vi "Option.vi"(8 "error in":errorcluster, 10 "Test Result In":T3, 11 "CalCfg File In":T2) -> (0 "error out":errorcluster, 1 "Pass":bool, 2 "Test Result Out":T3, 3 "CalCfg File Out":T2, 4 "String":string)   [LabVIEW 2020, in "GUCalibration2.lvlib"]
uses:
  GUCalibration2.lvlib
  Controls/Test Result.ctl
  Controls/Site Data Element.ctl
  Controls/Site Raw Data Element.ctl
  Controls/CalibrationOrCheck.ctl
  Utilities/Read Key Boolean.vi
  Utilities/Write Key Path.vi
  Utilities/Write Key Boolean.vi
panel:
  in  "Cal/Check":T1
  in  "GU Bench File Path":path
  in  "Cancel":bool
  in  "OK":bool
  in  "Offset File Path":path
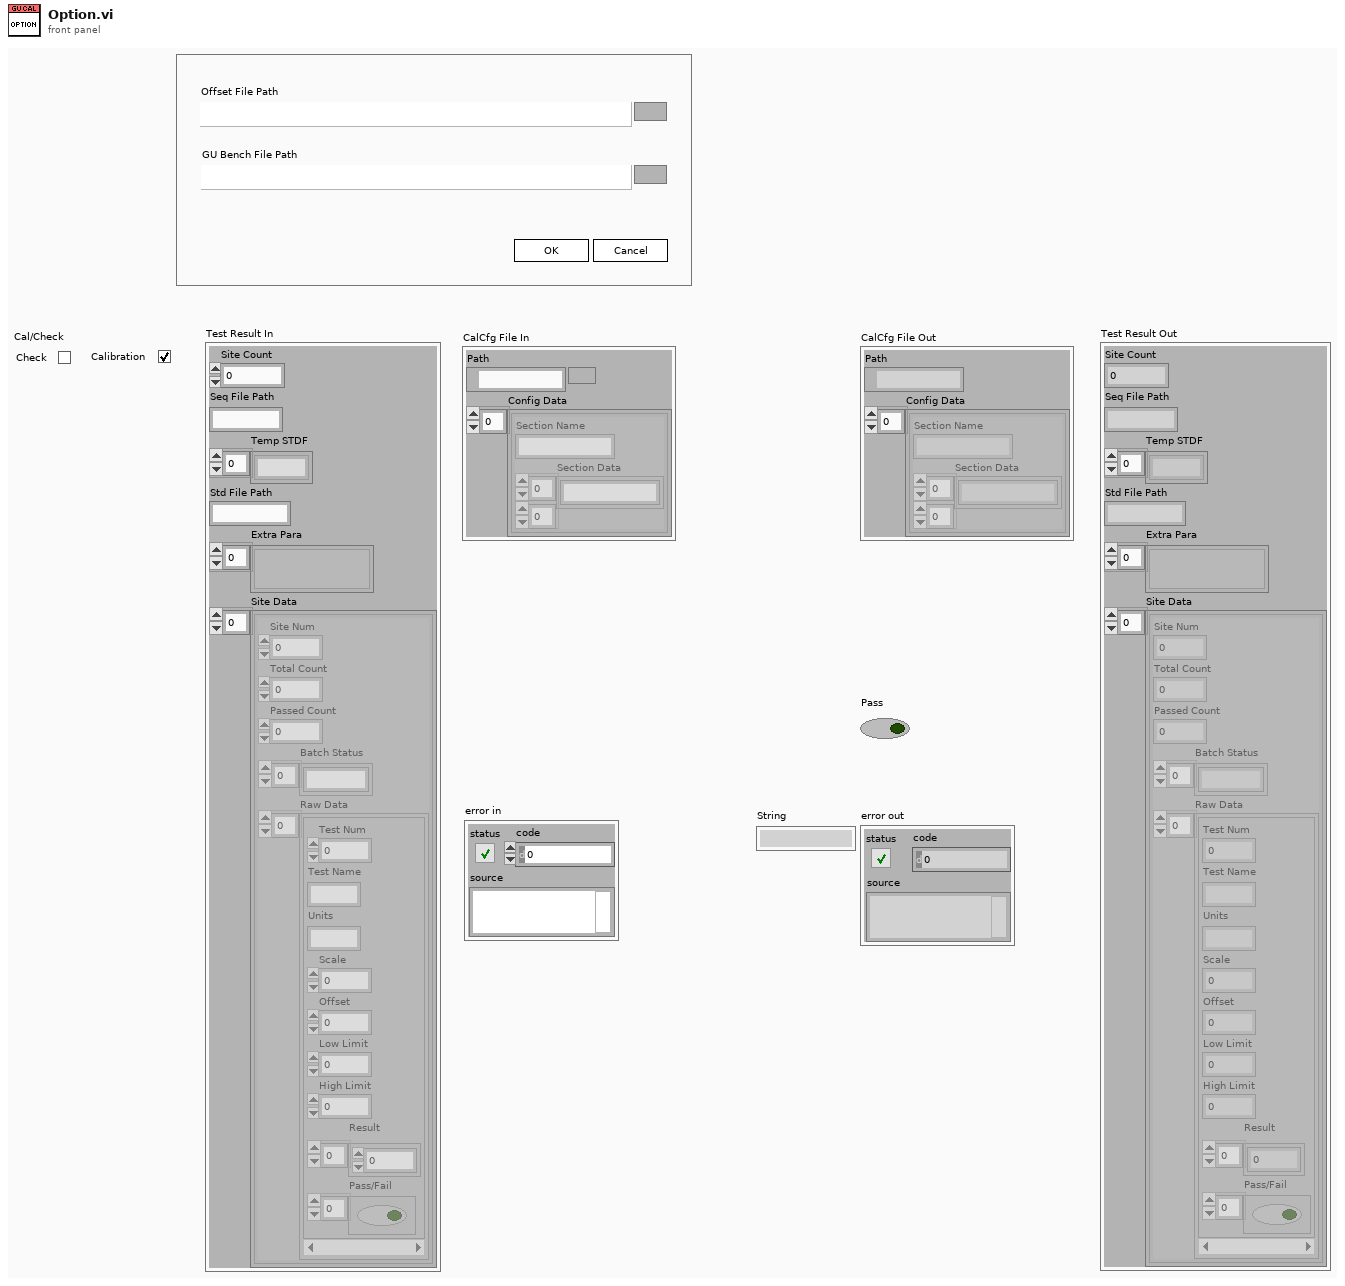
[diagram p1: front panel]
types:
  T1 = typedef "GUCalibration2.lvlib/CalibrationOrCheck.ctl" = enum32{"Calibration", "Check"}
  T2 = cluster{"Path":path, "Config Data":cluster{"Section Name":string, "Section Data":string[][]}[]}
  T3 = typedef "GUCalibration2.lvlib/Test Result.ctl" = cluster{"Site Count":i32, "Seq File Path":string, "Temp STDF":string[], "Std File Path":string, "Extra Para":variant[], "Site Data":T4[]}
  T4 = typedef "GUCalibration2.lvlib/Site Data Element.ctl" = cluster{"Site Num":i32, "Total Count":i32, "Passed Count":i32, "Batch Status":string[], "Raw Data":T5[]}
  T5 = typedef "GUCalibration2.lvlib/Site Raw Data Element.ctl" = cluster{"Test Num":u32, "Test Name":string, "Units":string, "Scale":i8, "Offset":dbl, "Low Limit":dbl, "High Limit":dbl, "Result":dbl[], "Pass/Fail":bool[]}
  T6 = cluster{"Section Name":string, "Section Data":string[][]}[]
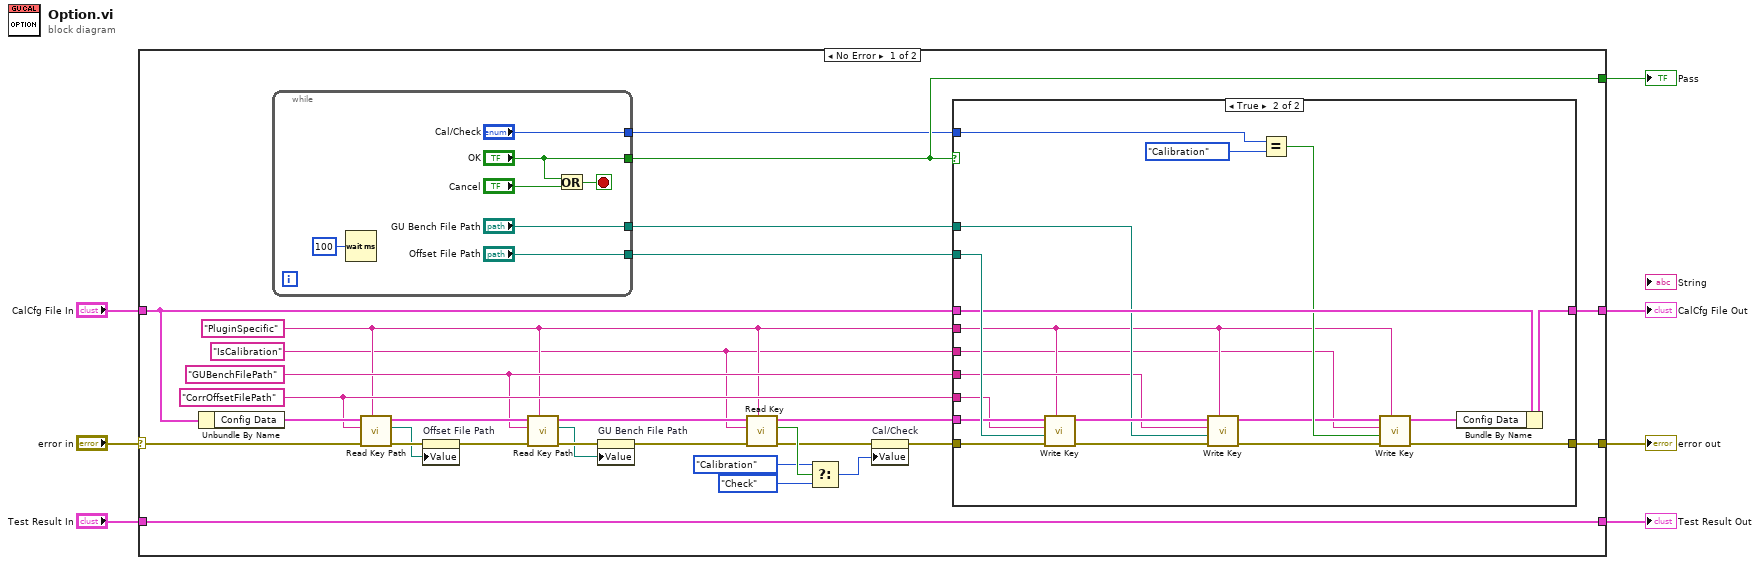
[diagram p0: block diagram]
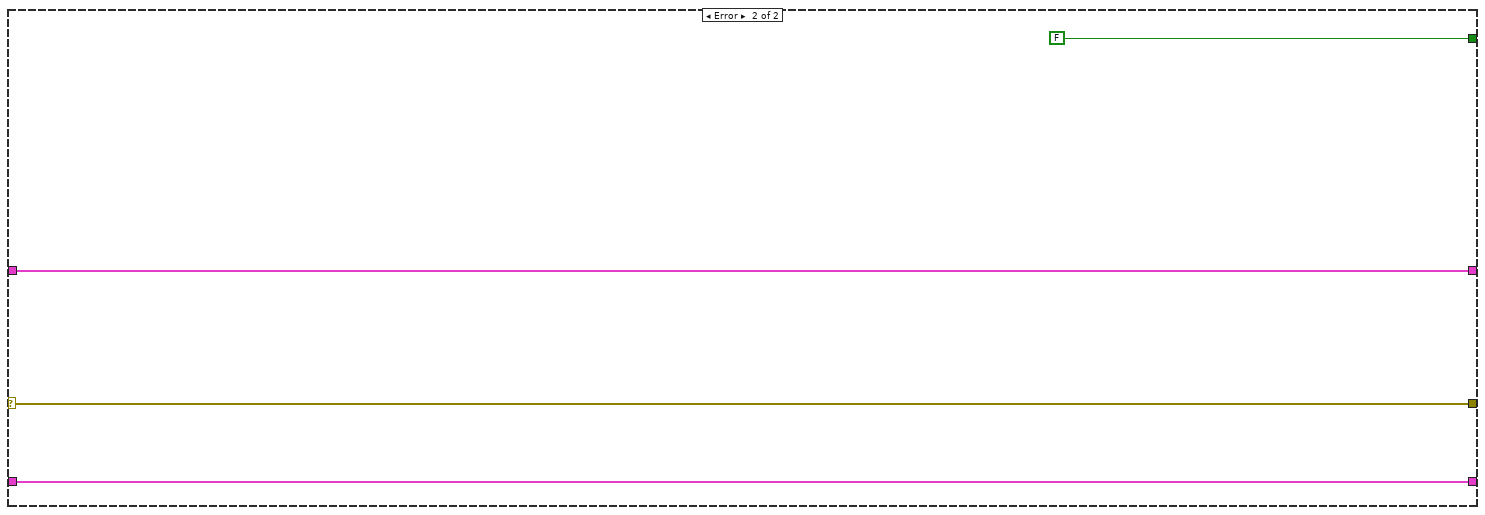
[diagram p3: hidden frame]
diagram:
  n1 = case shown="No Error" "error in" {
    selector: "error in" -> [w20 w68]
    tunnel: [w36 FALSE ("OK")] -> w7
    tunnel: [w34 w68] -> w6
    tunnel: [w33 w67] -> w5
    tunnel: "CalCfg File In" -> [w32 w67]
    tunnel: "Test Result In" -> [w21 w65]
    tunnel: [w21 w65] -> w2
    frame No Error {
      w15 = "GUBenchFilePath" ("Section Name")
      w10 = "IsCalibration" ("Section Name")
      w30 = "CorrOffsetFilePath" ("Section Name")
      w11 = "PluginSpecific" ("Section Name")
      n2 = Unbundle By Name(w32) -> ("Config Data"=w31:T6)
      n3 = while {
        tunnel: ["OK"] -> w36
        tunnel: ["Offset File Path"] -> w35
        tunnel: ["Cal/Check"] -> w27
        tunnel: ["GU Bench File Path"] -> w19
        stop <- w63 stop-if-true
        n4 = Wait (ms)(milliseconds to wait=u32 100) -> ()  [unwired: 1 out]
        n5 = Or(x="OK", y="Cancel") -> (x .or. y?=w63:bool)
      }
      n6 = call "Read Key Path.vi"("Section Name"=w11, "error in (no error)"=w20, "Key Names"=w30, "Config Data"=w31) -> ("error out"=w29:errorcluster, "Key Value out"=w28:path, "Config Data dup"=w18:T6)  [unwired: 3 in, 2 out]
      n7 = property on="Offset File Path" class="Path"(error in=w29, "Value"=w28) -> (error out=w16:errorcluster)  [unwired: 1 in, 1 out]
      n8 = call "Read Key Path.vi"("Section Name"=w11, "error in (no error)"=w16, "Key Names"=w15, "Config Data"=w18) -> ("error out"=w14:errorcluster, "Key Value out"=w12:path, "Config Data dup"=w17:T6)  [unwired: 3 in, 2 out]
      n9 = property on="GU Bench File Path" class="Path"(error in=w14, "Value"=w12) -> (error out=w13:errorcluster)  [unwired: 1 in, 1 out]
      n10 = call-poly "Read Key.vi"("Section Name"=w11, "error in (no error)"=w13, "Key Names"=w10, "Config Data"=w17) -> ("error out"=w24:errorcluster, "Key Value out"=w25:bool, "Config Data dup"=w26:T6)  [unwired: 3 in, 2 out]
      n11 = Select(t=CalibrationOrCheck."Calibration" ("Cal/Check"), s=w25, f=CalibrationOrCheck."Check" ("Cal/Check")) -> (s? t:f=w22:T1)
      n12 = property on="Cal/Check" class="RadioBtnsControl (strict)"(error in=w24, "Value"=w22) -> (error out=w23:errorcluster)  [unwired: 1 in, 1 out]
      n13 = case shown="True" w36 {
        tunnel: w35 -> [_ w56]
        tunnel: w23 -> [w38 w57]
        tunnel: [w38 w50] -> w34
        tunnel: w32 -> [w37 w55]
        tunnel: [w37 w54] -> w33
        tunnel: w26 -> [_ w53]
        tunnel: w30 -> [_ w52]
        tunnel: w27 -> [_ w49]
        tunnel: w19 -> [_ w43]
        tunnel: w15 -> [_ w42]
        tunnel: w11 -> [_ w41]
        tunnel: w10 -> [_ w40]
        frame False {
        }
        frame True {
          n14 = call-poly "Write Key.vi"("Section Name"=w41, "error in (no error)"=w57, "Key Value"=w56, "Key Name"=w52, "Config Data"=w53) -> ("error out"=w45:errorcluster, "Config Data dup"=w47:T6)  [unwired: 5 in]
          n15 = call-poly "Write Key.vi"("Section Name"=w41, "error in (no error)"=w45, "Key Value"=w43, "Key Name"=w42, "Config Data"=w47) -> ("error out"=w44:errorcluster, "Config Data dup"=w46:T6)  [unwired: 5 in]
          n16 = Equal?(x=w49, y=CalibrationOrCheck."Calibration" ("Cal/Check")) -> (x = y?=w48:bool)
          n17 = call-poly "Write Key.vi"("Section Name"=w41, "error in (no error)"=w44, "Key Value"=w48, "Key Name"=w40, "Config Data"=w46) -> ("error out"=w50:errorcluster, "Config Data dup"=w51:T6)  [unwired: 5 in]
          n18 = Bundle By Name(cluster=w55, "Config Data"=w51) -> (w54:T2)
        }
      }
    }
    frame Error {
    }
  }
  "error out" <- w6
  "Pass" <- w7
  "Test Result Out" <- w2
  "CalCfg File Out" <- w5
